vi "Read Section Names.vi"(8 "error in (no error)":errorcluster, 11 "ODBC-Interface in":refnum<class "ODBC-Interface.lvclass">) -> (0 "error out":errorcluster, 1 "Section Names":string[](array[string]), 2 "Section Classes":path[](array[path]), 3 "ODBC-Interface out":refnum<class "ODBC-Interface.lvclass">)   [LabVIEW 2012, in "DB-Configuration.lvlib" / "ODBC-Interface.lvclass"]
doc: "Read available sections and pathes to corresponding derived class of Sections.lvclass."
uses:
  ODBC-Interface.lvclass
  ODBC-Interface.lvclass/ODBC-Interface.ctl
  <vilib>/addons/database/Connection.llb/Conn Execute.vi
  <vilib>/addons/database/Recordset.llb/Rec Fetch Recordset Data (R).vi
  <vilib>/addons/database/Recordset.llb/Rec Destroy - Connection.vi
  <vilib>/addons/database/_DB Variant To Data/Database Variant To Data.xnode
  DB-Configuration.lvlib
  <vilib>/addons/database/NI_Database_API.lvlib
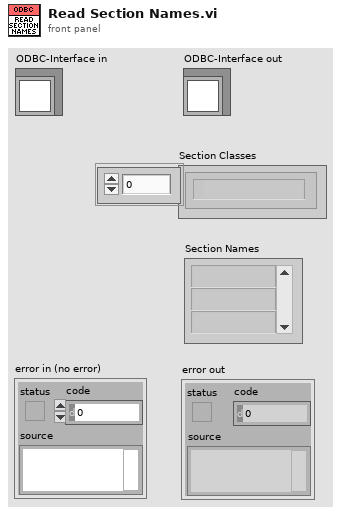
[diagram p1: front panel]
types:
  T1 = typedef "NI_Database_API.lvlib/Conn ObjectReference.ctl" = refnum<k1>
  T2 = typedef "NI_Database_API.lvlib/Rec ObjectReference.ctl" = refnum<k1>
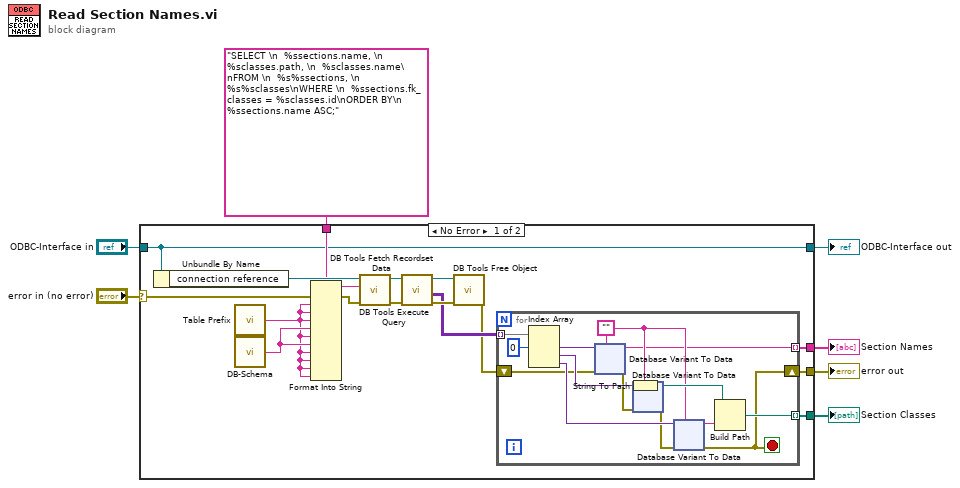
[diagram p0: block diagram]
diagram:
  n1 = case shown="No Error" "error in (no error)" {
    selector: "error in (no error)" -> [w9 w136]
    tunnel: "ODBC-Interface in" -> [w8 w137]
    tunnel: "SELECT \n  %ssections.name, \n  %sclasses.path, \n  %sclasses.name\nFROM \n  %s%ssections, \n  %s%sclasses\nWHERE \n  %ssections.fk_classes = %sclasses.id\nORDER BY\n  %ssections.name ASC;" -> [w23 _]
    tunnel: [w12 _] -> w5
    tunnel: [w11 w136] -> w4
    tunnel: [w10 _] -> w3
    tunnel: [w8 w137] -> w1
    frame No Error {
      n2 = Unbundle By Name(w8) -> ("connection reference"=w24:T1)
      n3 = call "Table Prefix.vi"() -> ("DB Table Prefix"=w20:string)
      n4 = call "DB-Schema.vi"() -> ("DB Schema (public.)"=w21:string)
      n5 = Format Into String(format string=w23, error in=w9, w20, w20, w20, w21, w20, w21, w20, w20, w20, w20) -> (resulting string=w22:string, error out=w19:errorcluster)  [unwired: 1 in]
      n6 = call-poly <vilib>:"DB Tools Execute Query.vi"("error in (no error)"=w19, "SQL query"=w22, "connection reference"=w24) -> ("error out"=w17:errorcluster, "recordset reference"=w18:T2)  [unwired: 5 in]
      n7 = call-poly <vilib>:"DB Tools Fetch Recordset Data.vi"("error in (no error)"=w17, "recordset reference"=w18) -> ("error out"=w16:errorcluster, "recordset data"=w14:variant[][], "recordset reference out"=w15:T2)  [unwired: 3 in]
      n8 = call-poly <vilib>:"DB Tools Free Object.vi"("error in (no error)"=w16, "recordset reference"=w15) -> ("error out"=w13:errorcluster)  [unwired: 8 in, 1 out]
      n9 = for {
        tunnel: w14 -> [w39] mode=indexing
        shift-right: [w25] -> w11
        shift-left: w13 -> [w31]
        tunnel: [w27] -> w12 mode=indexing
        tunnel: [w26] -> w10 mode=indexing
        stop <- w25 stop-if-true
        w28 = ""
        n10 = Index Array(array=w39, index #1=0 ("index")) -> (element #1=w37:variant, element #2=w36:variant, element #3=w35:variant)  [unwired: 2 in]
        n11 = xnode "Database Variant To Data"("database variant"=w37, "error in (no error)"=w31, "type"=w28) -> ("data"=w27:string, "error out"=w30:errorcluster)
        n12 = xnode "Database Variant To Data"("database variant"=w36, "error in (no error)"=w30, "type"=w28) -> ("data"=w34:string, "error out"=w29:errorcluster)
        n13 = String To Path(string=w34) -> (path=w33:path)
        n14 = xnode "Database Variant To Data"("database variant"=w35, "error in (no error)"=w29, "type"=w28) -> ("data"=w32:string, "error out"=w25:errorcluster)
        n15 = Build Path(base path=w33, name or relative path=w32) -> (appended path=w26:path)
      }
    }
    frame Error {
    }
  }
  "error out" <- w4
  "ODBC-Interface out" <- w1
  "Section Names" <- w5
  "Section Classes" <- w3
